vi "disconnectSubDataSubscribe.vi"(8 "error in (no error)":errorcluster, 11 "MiddlewareSALThisComponent in":refnum<class "MiddlewareSALThisComponent.lvclass">) -> (0 "error out":errorcluster, 3 "MiddlewareSALThisComponent out":refnum<class "MiddlewareSALThisComponent.lvclass">)   [LabVIEW 2016, in "MiddlewareSALThisComponent.lvclass"]
uses:
  MiddlewareSALThisComponent.lvclass
  ProgrammaticInitialization/ProgrammaticInitialization.lvclass
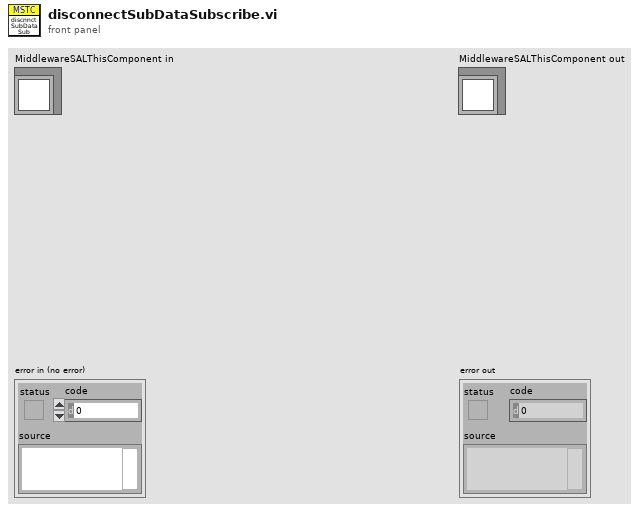
[diagram p1: front panel]
types:
  T1 = typedef "ProgrammaticInitialization.lvclass/cmdsToSubscribeDL.ctl" = string[]
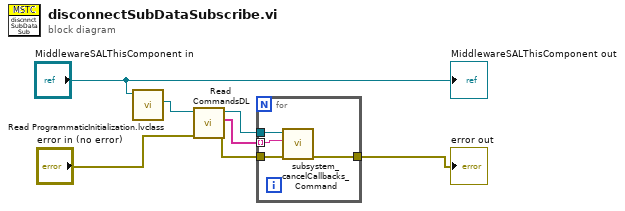
[diagram p0: block diagram]
diagram:
  n1 = call-dynamic "Read ProgrammaticInitialization.lvclass.vi"("MiddlewareSALThisComponent in"="MiddlewareSALThisComponent in") -> ("ProgrammaticInitialization.lvclass"=w6:refnum<class "ProgrammaticInitialization.lvclass">)  [unwired: 8 in, 2 out]
  n2 = call-dynamic "Read CommandsDL.vi"("error in (no error)"="error in (no error)", "ProgrammaticInitialization in"=w6) -> ("error out"=w2:errorcluster, "CommandsDL"=w3:T1, "ProgrammaticInitialization out"=w4:refnum<class "ProgrammaticInitialization.lvclass">)  [unwired: 7 in]
  n3 = for {
    tunnel: w4 -> [w11]
    tunnel: w3 -> [w10] mode=indexing
    tunnel: w2 -> [w9]
    tunnel: [w8] -> w1
    n4 = call "subsystem_cancelCallbacks_Command.vi"("error in (no error)"=w9, "topic"=w10, "ProgrammaticInitialization in"=w11) -> ("error out"=w8:errorcluster)  [unwired: 7 in, 1 out]
  }
  "error out" <- w1
  "MiddlewareSALThisComponent out" <- "MiddlewareSALThisComponent in"
